vi "remove control module.vi"(7 "engine in":refnum<class "engine configuration.lvclass">, 8 "error in":errorcluster, 9 "owner id":string, 10 "name":string, 11 "user module configuration in":refnum<class "TEST CONFIGURATION.lvclass">) -> (0 "error out":errorcluster, 3 "user module configuration out":refnum<class "TEST CONFIGURATION.lvclass">, 5 "engine out":refnum<class "engine configuration.lvclass">)   [LabVIEW 2013, in "configuration tests.lvlib" / "TEST CONFIGURATION.lvclass"]
uses:
  TEST CONFIGURATION.lvclass
  <vilib>/NI/Module Execution Interface/Engine Configuration/engine configuration.lvclass
  TEST CONFIGURATION.lvclass/TEST CONFIGURATION.ctl
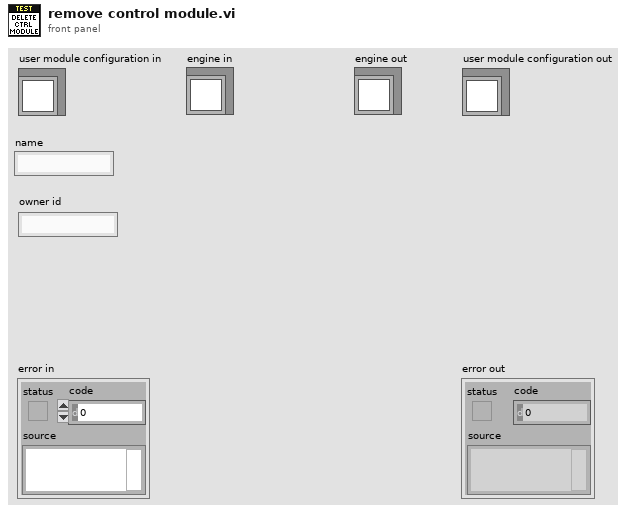
[diagram p1: front panel]
types:
  T1 = typedef "configuration tests.lvlib/TEST CONFIGURATION.lvclass/control module configuration.ctl" = cluster{"name":string, "setpoint":refnum<class "TBM channel.lvclass">, "process variable":refnum<class "TBM channel.lvclass">, "output":refnum<class "TBM channel.lvclass">, "gains":T2, "output range":cluster{"output high":dbl, "output low":dbl}}
  T2 = typedef "configuration tests.lvlib/TEST CONFIGURATION.lvclass/gains.ctl" = cluster{"Kp":dbl, "Ki":dbl, "Kd":dbl}
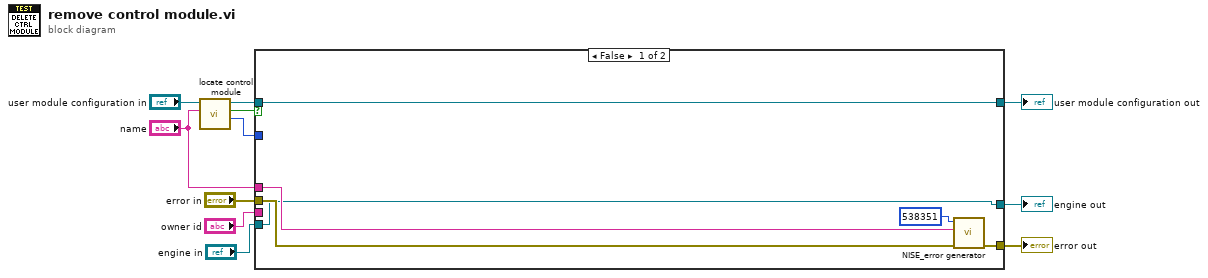
[diagram p0: block diagram]
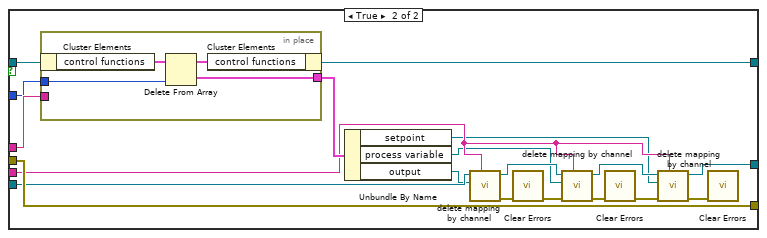
[diagram p2: hidden frame]
diagram:
  n1 = call "locate control module.vi"("name"="name", "user module configuration in"="user module configuration in") -> ("index"=w4:i32, "found"=w9:bool, "user module configuration out"=w10:refnum<class "TEST CONFIGURATION.lvclass">)  [unwired: 6 in, 1 out]
  n2 = case shown="False" w9 {
    tunnel: w10 -> [w14 w36]
    tunnel: "error in" -> [w17 w28]
    tunnel: [w15 w28] -> w7
    tunnel: [w14 w35] -> w6
    tunnel: "name" -> [w13 w34]
    tunnel: w4 -> [_ w33]
    tunnel: "engine in" -> [w12 w25]
    tunnel: "owner id" -> [_ w22]
    tunnel: [w12 w21] -> w1
    frame False {
      n3 = call <vilib>:"NISE_error generator.vi"("error in"=w17, "append error message"=w13, "error code (0)"=538351) -> ("error out"=w15:errorcluster)  [unwired: 6 in]
    }
    frame True {
      n4 = in-place {
        in-place-border: w34 -> [_]
        in-place-border: w33 -> [w38]
        in-place-border: [w37] -> w32
        n5 = in-place-cluster #1(w36) -> ("control functions"=w40:T1[])
        n6 = Delete From Array(array=w40, index=w38) -> (deleted portion=w37:T1, array with subset deleted=w39:T1[])  [unwired: 1 in]
        n7 = in-place-cluster #1("control functions"=w39) -> (w35:refnum<class "TEST CONFIGURATION.lvclass">)
      }
      n8 = Unbundle By Name(w32) -> ("setpoint"=w20:refnum<class "TBM channel.lvclass">, "process variable"=w19:refnum<class "TBM channel.lvclass">, "output"=w18:refnum<class "TBM channel.lvclass">)
      n9 = call <vilib>:"delete mapping by channel.vi"("owner ID"=w22, "channel"=w18, "engine configuration in"=w25) -> ("error out"=w31:errorcluster, "engine configuration out"=w24:refnum<class "engine configuration.lvclass">)  [unwired: 7 in]
      n10 = call <vilib>:"Clear Errors.vi"("error in (no error)"=w31) -> ("error out"=w27:errorcluster)  [unwired: 6 in]
      n11 = call <vilib>:"delete mapping by channel.vi"("owner ID"=w22, "error in"=w27, "channel"=w19, "engine configuration in"=w24) -> ("error out"=w30:errorcluster, "engine configuration out"=w23:refnum<class "engine configuration.lvclass">)  [unwired: 6 in]
      n12 = call <vilib>:"Clear Errors.vi"("error in (no error)"=w30) -> ("error out"=w26:errorcluster)  [unwired: 6 in]
      n13 = call <vilib>:"delete mapping by channel.vi"("owner ID"=w22, "error in"=w26, "channel"=w20, "engine configuration in"=w23) -> ("error out"=w29:errorcluster, "engine configuration out"=w21:refnum<class "engine configuration.lvclass">)  [unwired: 6 in]
      n14 = call <vilib>:"Clear Errors.vi"("error in (no error)"=w29) -> ()  [unwired: 6 in, 1 out]
    }
  }
  "error out" <- w7
  "user module configuration out" <- w6
  "engine out" <- w1
